vi "chaosui-crest-cmd.vi"(7 "args":string, 9 "cmd":string, 10 "cuname":string) -> ()   [LabVIEW 2014, in "chaosui-crest.lvlib"]
doc: "int chaos_crest_cu_cmd(chaos_crest_handle_t h,const char*cuname,const char*cmd,const char* args);"
uses:
  chaosui-crest.lvlib
  <vilib>/httpClient/ClientHandle.ctl
  <vilib>/httpClient/LabVIEWHTTPClient.lvlib
panel:
  out "nok":i32
  in  "handleConnection":T2
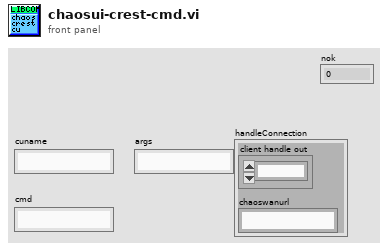
[diagram p1: front panel]
types:
  T1 = typedef "LabVIEWHTTPClient.lvlib/ClientHandle.ctl" = refnum<k1>
  T2 = cluster{"client handle out":T1, "chaoswanurl":string}
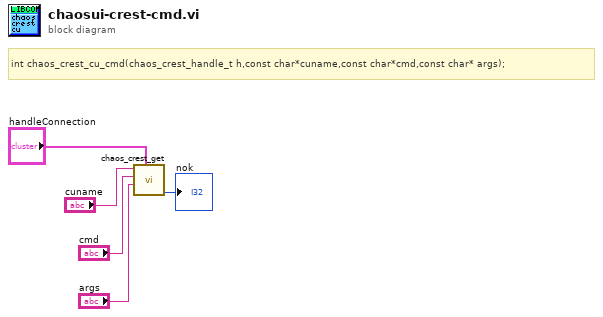
[diagram p0: block diagram]
diagram:
  # "int chaos_crest_cu_cmd(chaos_crest_handle_t h,const char*cuname,const char*cmd,const char* args);"
  n1 = call "chaos_crest_get.vi"("cuname"="cuname", "cmd"="cmd", "args"="args", "handleConnection"="handleConnection") -> ("nok"=→"nok":i32)  [unwired: 4 in, 2 out]
